vi "获取简易流程名称API.vi"(8 "error in (no error)":errorcluster, 11 "参数下拉列表":u16) -> (0 "error out":errorcluster, 3 "字符串与值[]":T1)   [LabVIEW 2016, in "斯坦道总磷总氮.lvlib"]
uses:
  <vilib>/Utility/miscctls.llb/LVStringsAndValuesArrayTypeDef_U16.ctl
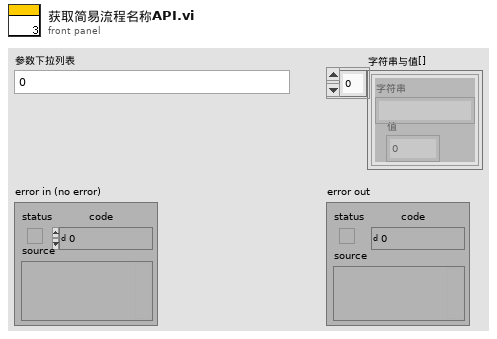
[diagram p1: front panel]
types:
  T1 = typedef "LVStringsAndValuesArrayTypeDef_U16.ctl" = cluster{"String":string, "Value":u16}[]
  T2 = typedef "SingleStepTestV3.lvlib/SingleStepTestV3.lvclass/仪器版本.ctl" = enum16{"V3.1版", "V4版", "V3版", "V4.2版"}
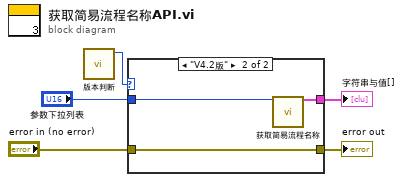
[diagram p0: block diagram]
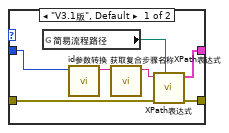
[diagram p2: hidden frame]
diagram:
  n1 = call "版本判断.vi"() -> ("仪器版本"=w5:T2)  [unwired: 11 in]
  n2 = case shown="\"V4.2版\"" w5 {
    tunnel: [w10 w14] -> w1
    tunnel: "参数下拉列表" -> [w9 w15]
    tunnel: [w7 w13] -> w2
    tunnel: "error in (no error)" -> [w6 w13]
    frame "V3.1版", Default {
      n3 = global read "总磷总氮断电保存全局变量.vi" "简易流程路径"() -> (w11:path)
      n4 = call "id参数转换.vi"("id"=w9) -> ("table输出"=w8:string)  [unwired: 9 in, 1 out]
      n5 = call "获取复合步骤名称XPath表达式.vi"("查询参数"=w8) -> ("Union"=w12:string)  [unwired: 10 in]
      n6 = call "XPath表达式.vi"("添加的路径"=w11, "error in (no error)"=w6, "XPath expression"=w12) -> ("error out"=w7:errorcluster, "字符串与值[]"=w10:T1)  [unwired: 7 in]
    }
    frame "V4.2版" {
      n7 = call "获取简易流程名称.vi"("参数下拉列表"=w15) -> ("字符串与值[]"=w14:T1)  [unwired: 18 in]
    }
  }
  "error out" <- w2
  "字符串与值[]" <- w1
